vi "I2C Utility Example EEPROM Repeat.vi"() -> ()   [LabVIEW 2020]
panel:
  out "I2C COM Error":string="No Error"
  out "Acks Received":dbl
  out "I2C_ACKS (Repeated)":u32[](array[numeric]) format="%x"
  out "I2C_READ_DATA (Repeated)":u8[][](array[numeric]) format="%x"
  in  "Tab Control":enum32{"Write", "Write/Read"}(tab)=enum."Write/Read"
  out "I2C_READ_DATA (Write)":u8[](array[numeric]) format="%x"
  in  "Num Repeat (Write)":i32
  in  "I2C_NUM_BYTES_RX (Write)":i32
  in  "I2C_WRITE_DATA (Write)":i32[](array[numeric])=[0, 222, 173, 190, 239, 1, 2, 3, 4, 5, 6, 7, 222, 173, 190, 239] format="%x"
  out "I2C_READ_DATA (read)":u8[](array[numeric]) format="%x"
  in  "Num Repeat (Read)":i32=4
  in  "I2C_NUM_BYTES_RX (Read)":i32=15
  in  "I2C_WRITE_DATA (Read)":i32[](array[numeric])=[0] format="%x"
  in  "I2C_SLAVE_ADDRESS":i32=80
  in  "I2C_OPTIONS":i32
  in  "I2C_SPEED_THROTTLE":i32
  in  "I2C_SCL_DIONUM":i32=1
  in  "I2C_SDA_DIONUM":i32
  out "Error String":string="No Error"
  out "error out":errorcluster
  out "ConnectionType Out":i32
  out "DeviceType Out":i32
  in  "Identifier":string="LJM_idANY"
  in  "ConnectionType":string="LJM_ctANY"
  in  "DeviceType":string="LJM_dtANY"
  # "Before running this program:\n1. Attach a LJTick-DAC to FIO0 and FIO1\n2. Configure Device Opening Settings (DeviceType, ConnectionType, and Identifier)\n3. Configure I2C Settings (I2C_SDA_DIONUM, I2C_SCL_DIONUM, I2C_SPEED_THROTTLE, I2C_OPTIONS, I2C_SLAVE_ADDRESS)\n4. Select appropriate tab for I2C Functionality, described below.  Either \"Write\" or \"Write/Read\"  the visible tab is the mode \n    that will be executed.\n5. Run the .vi by either 'ctrl+r' or by pressing the \"Run\" button.\n\nThis program interfaces with the Microchip 24C01C EEPROM built into the LJTick-DAC, it has a Slave Address of 0x50 or d80.  \nThis program lets you write and read data to/from the EEPROM.  It uses the \"I2C Utility.vi\" to configure and control a LabJack T7's \nI2C functionality.   It is important to note that this EEPROM lets you perform page read's and writes of 1-15 bytes of data.  This\nprogram does not check that limitation and report an error, you have been warned!\n\nWrite: \nBy default selecting this tab lets you write 0-15 bytes of data to the EEPROM starting at page (PageNum).  It configures the LabJack to:\n1. Send a Start I2C command\n2. Send the Slave Address followed by a write bit (0)\n3. Wait for an Ack from the EEPROM\n4. Write the remaining bytes of data while waiting for Acks.\n\nThings that can be configured:\n1. You can configure the starting Page to write to by changing the PageNum value in the \"I2C_WRITE_DATA (Write) array.\n2. You can configure how many values to write by declaring/deleting elements from the \"I2C_WRITE_DATA (Write) array.\n    Right click on array, \"Data Operations\"->\"Delete Element\" or \"Insert Element Before\".\n3. You can configure how many bytes are read after data is written.  Is 0  default in this mode so that data is only written.\n4.  You can configure how many times this operation is repeated, by changing the \"Num Repeat (Write)\" value.  Sends\n    \"I2C_GO\" and \"I2C_ACKS\" requests to the device.  Be careful, EEPROMS only support a limited number of writes to each page!\n\nWrite/Read:\nBy default selecting this tab lets you read 0-15 bytes of data from the EEPROM starting at page (PageNum).  It configures the LabJack to:\n1. Send a Start I2C command.\n2. Send the Slave Address followed by a write bit (0) & wait for an ACK from the EEPROM.\n3. Write the starting PageNum to read from & wait for an ACK from the EEPROM.\n4. Perform configured start/restart condition (configurable by the I2C_OPTIONS value).\n5. Send the Slave Address followed by a read bit (1) & wait for an ACK from the EEPROM.\n6. Begin receiving values from the EEPROM & sending ACK's back after each byte is received.\n\nThings that can be configured:\n1. You can configure the starting Page to read from by changing the PageNum value in the \"I2C_WRITE_DATA (Read) array.\n2. You can configure how many values to write by declaring/deleting elements from the \"I2C_WRITE_DATA (Read) array.\n    Right click on array, \"Data Operations\"->\"Delete Element\" or \"Insert Element Before\".  \n    By default this element is one value long and 0 to configure reading starting at page 0.\n3. You can configure how many bytes are read after the PageNum is written.  Is 15  default in this mode to indicate 15 bytes \n    of data need to be read after configuring the EEPROM.\n4.  You can configure how many times this operation is repeated, by changing the \"Num Repeat (Write)\" value.  Sends\n    \"I2C_GO\" (to start the I2C request), \"I2C_ACKS\" (to read the number of ACKS read by the LabJack), and \"I2C_READ_DATA\"\n    (to read the data read by the LabJack requests to the device)."
  # "I2C Functionality (Select a tab)"
  # "Device Opening Settings"
  # "Data [0]"
  # "Data [1]"
  # "Data [2]"
  # "Data [3]"
  # "..."
  # "I2C Settings"
  # "Configures the FIO channel that the \nSDA signal should appear on."
  # "Configures the FIO channel that the \nSDA signal should appear on."
  # "Configures the I2C Clock Speed\n (frequency)"
  # "Configures the I2C options"
  # "..."
  # "Data [14]"
  # "Configure the slave address to be sent \nat the start of each data transfer"
  # "Errors:"
  # "PageNum"
  # "Data [0]"
  # "Data [0]"
  # "Data [1]"
  # "Data [1]"
  # "Data [2]"
  # "Data [2]"
  # "Data [3]"
  # "Data [3]"
  # "..."
  # "..."
  # "..."
  # "..."
  # "Data [14]"
  # "Data [14]"
  # "PageNum"
  # "Data [0]"
  # "Data [0]"
  # "Data [1]"
  # "Data [1]"
  # "Data [2]"
  # "Data [2]"
  # "Data [3]"
  # "Data [3]"
  # "..."
  # "..."
  # "..."
  # "..."
  # "Data [14]"
  # "Data [14]"
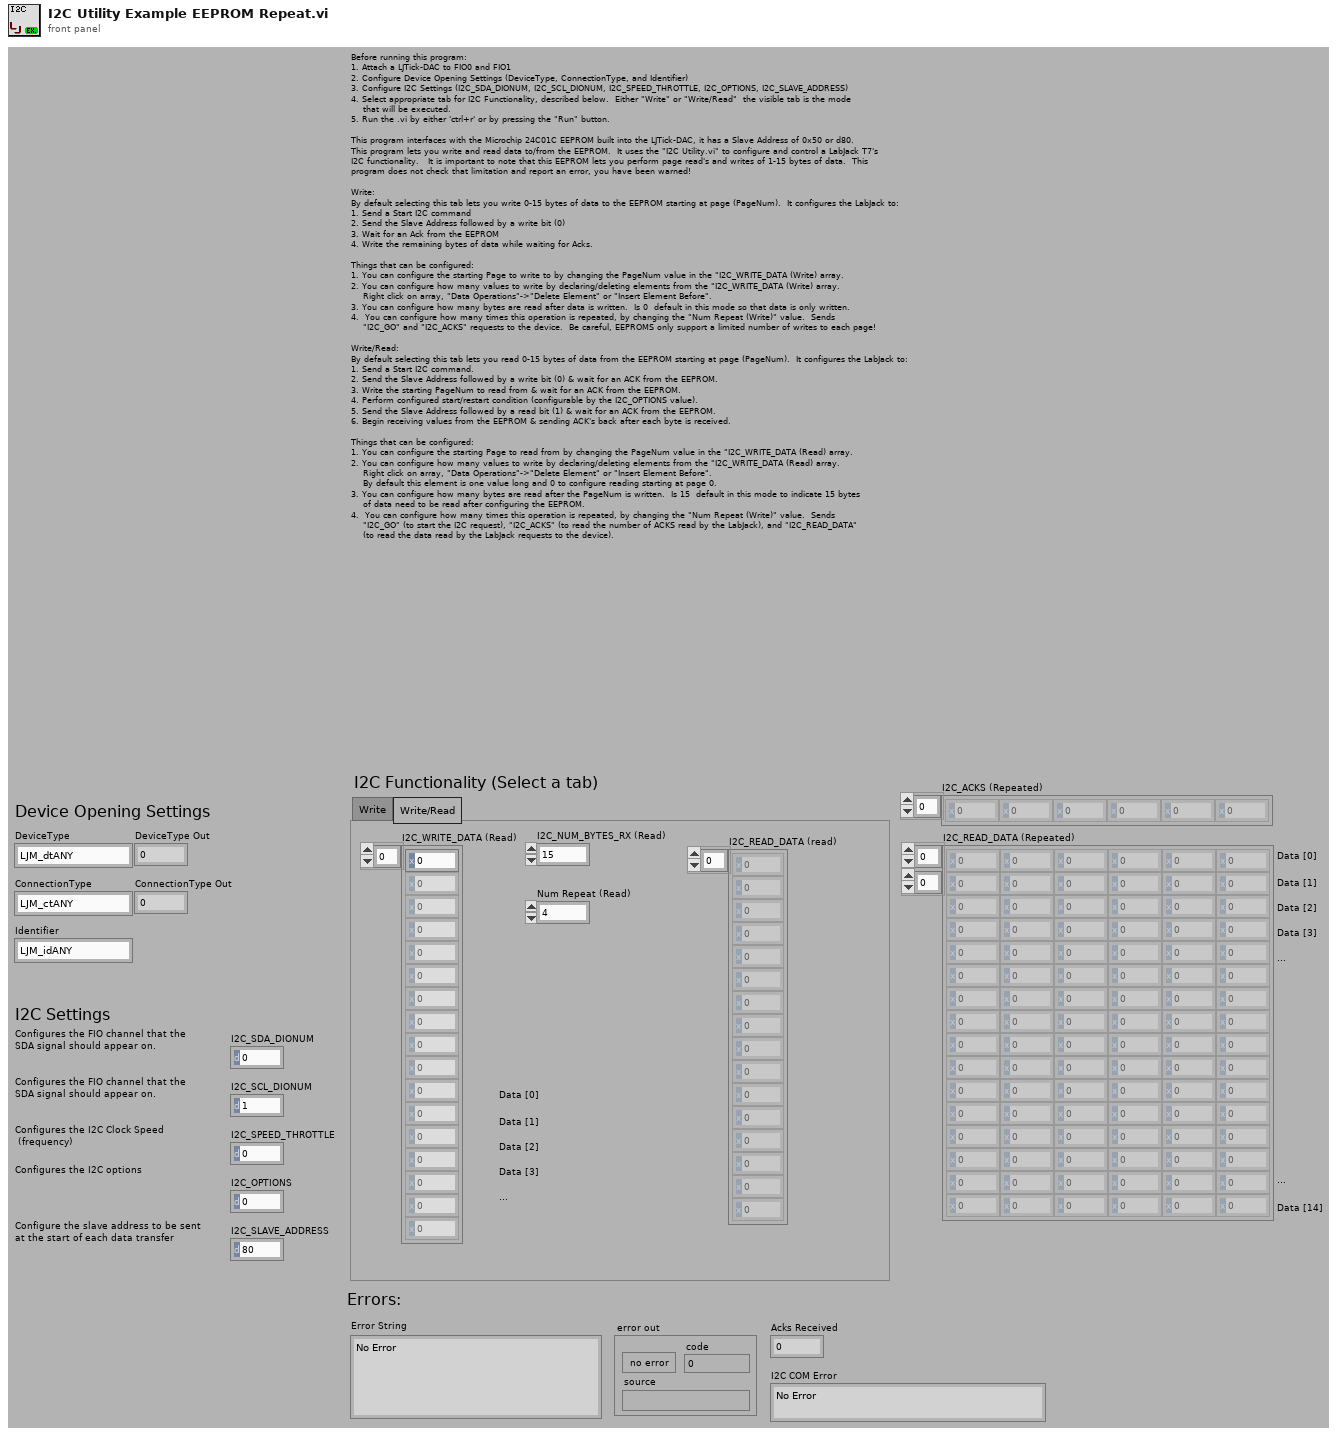
[diagram p1: front panel]
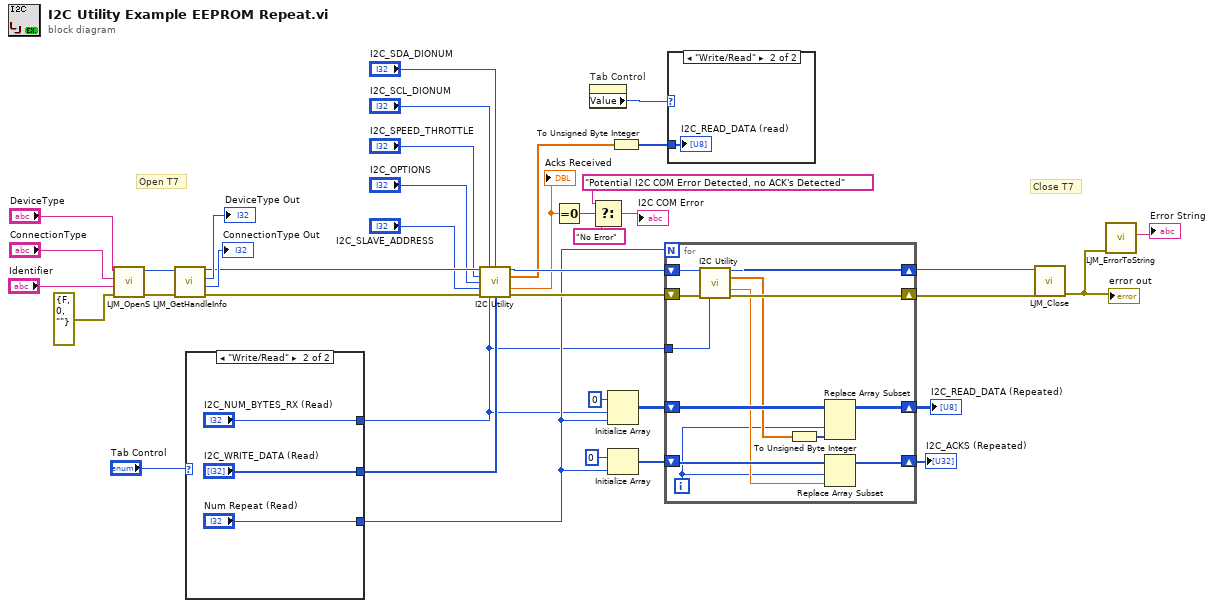
[diagram p0: block diagram]
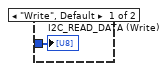
[diagram p2: hidden frame]
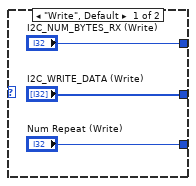
[diagram p3: hidden frame]
diagram:
  # "Close T7"
  # "Open T7"
  n1 = call "LJM_OpenS.vi"("error in"=errorcluster {"status"=FALSE, "code"=0, "source"=""} ("error in (no error)"), "Identifier"="Identifier", "ConnectionType"="ConnectionType", "DeviceType"="DeviceType") -> ("error out"=w38:errorcluster, "Handle"=w37:i32)  [unwired: 6 in]
  n2 = call "LJM_GetHandleInfo.vi"("error in"=w38, "Handle In"=w37) -> ("error out"=w28:errorcluster, "ConnectionType"=→"ConnectionType Out":i32, "DeviceType"=→"DeviceType Out":i32, "Handle Out"=w29:i32)  [unwired: 2 in, 4 out]
  n3 = case shown="\"Write/Read\"" "Tab Control" {
    tunnel: ["I2C_NUM_BYTES_RX (Write)" "I2C_NUM_BYTES_RX (Read)"] -> w6
    tunnel: ["I2C_WRITE_DATA (Write)" "I2C_WRITE_DATA (Read)"] -> w17
    tunnel: ["Num Repeat (Write)" "Num Repeat (Read)"] -> w7
    frame "Write", Default {
    }
    frame "Write/Read" {
    }
  }
  n4 = call "I2C Utility.vi"("Handle In"=w29, "I2C_SDA_DIONUM"="I2C_SCL_DIONUM", "I2C_SCL_DIONUM"="I2C_SDA_DIONUM", "I2C_SPEED_THROTTLE"="I2C_SPEED_THROTTLE", "I2C_OPTIONS"="I2C_OPTIONS", "I2C_SLAVE_ADDRESS"="I2C_SLAVE_ADDRESS", "error in"=w28, "I2C_NUM_BYTES_RX"=w6, "I2C_WRITE_DATA"=w17) -> ("Handle Out"=w22:i32, "Data Read"=w15:dbl[], "Acks Received"=w5:dbl, "error out"=w21:errorcluster)  [unwired: 2 in, 1 out]
  "Acks Received" <- w5
  n5 = Equal To 0?(x=w5) -> (x = 0?=w4:bool)
  n6 = property on="Tab Control" class="TabCtl (strict)"() -> ("Value"=w16:enum32{"Write", "Write/Read"})  [unwired: 2 in, 2 out]
  n7 = Select(t="Potential I2C COM Error Detected, no ACK's Detected", s=w4, f="No Error") -> (s? t:f=→"I2C COM Error":string)
  n8 = Initialize Array(u8 0, w6, w7) -> (w12:u8[][])
  n9 = Initialize Array(u32 0 ("element"), w7) -> (w10:u32[])
  n10 = To Unsigned Byte Integer(number=w15) -> (unsigned 8bit integer=w14:u8[])
  n11 = for {
    N: w7 -> [_]
    shift-right: [w56] -> w20
    shift-left: w22 -> [w58]
    shift-right: [w55] -> w19
    shift-left: w21 -> [w57]
    shift-right: [w54] -> w9
    shift-left: w12 -> [w53]
    shift-right: [w49] -> w8
    shift-left: w10 -> [w50]
    tunnel: w6 -> [w46]
    i -> [w47]
    n12 = call "I2C Utility.vi"("Handle In"=w58, "error in"=w57, "I2C_NUM_BYTES_RX"=w46) -> ("Handle Out"=w56:i32, "Data Read"=w52:dbl[], "Acks Received"=w48:dbl, "error out"=w55:errorcluster)  [unwired: 8 in, 1 out]
    n13 = To Unsigned Byte Integer(number=w52) -> (unsigned 8bit integer=w51:u8[])
    n14 = Replace Array Subset(array=w53, new element=w51, index (col)=w47) -> (w54:u8[][])  [unwired: 1 in]
    n15 = Replace Array Subset(array=w50, new element=w48, index=w47) -> (w49:u32[])
  }
  "I2C_READ_DATA (Repeated)" <- w9
  "I2C_ACKS (Repeated)" <- w8
  n16 = case shown="\"Write/Read\"" w16 {
    tunnel: w14 -> [w59 w60]
    frame "Write", Default {
      "I2C_READ_DATA (Write)" <- w59
    }
    frame "Write/Read" {
      "I2C_READ_DATA (read)" <- w60
    }
  }
  n17 = call "LJM_Close.vi"("error in"=w19, "Handle"=w20) -> ("error out"=w31:errorcluster)  [unwired: 9 in]
  "error out" <- w31
  n18 = call "LJM_ErrorToString.vi"("error in"=w31) -> ("String"=→"Error String":string)  [unwired: 10 in]
